vi "reverse calibration.vi"(9 "STAMP intercept":dbl, 10 "STAMP slope":dbl=1.0, 11 "RPM Calibration in":T1) -> (3 "RPM Calibration":T1)   [LabVIEW 2015]
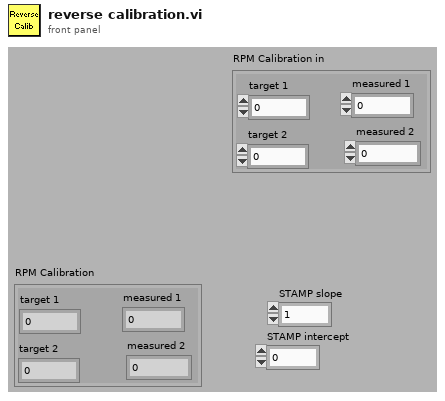
[diagram p1: front panel]
types:
  T1 = cluster{"target 1":dbl, "target 2":dbl, "measured 1":dbl, "measured 2":dbl}
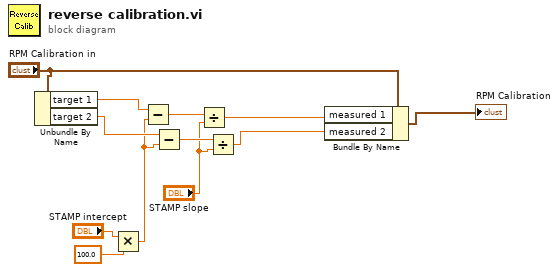
[diagram p0: block diagram]
diagram:
  n1 = Unbundle By Name("RPM Calibration in") -> ("target 1"=w8:dbl, "target 2"=w7:dbl)
  n2 = Multiply(x="STAMP intercept", y=100.0) -> (x*y=w6:dbl)
  n3 = Subtract(x=w8, y=w6) -> (x-y=w5:dbl)
  n4 = Subtract(x=w7, y=w6) -> (x-y=w4:dbl)
  n5 = Divide(x=w5, y="STAMP slope") -> (x/y=w2:dbl)
  n6 = Divide(x=w4, y="STAMP slope") -> (x/y=w1:dbl)
  n7 = Bundle By Name(cluster="RPM Calibration in", "measured 1"=w2, "measured 2"=w1) -> (→"RPM Calibration":T1)
